vi "HC-SR04 Trigg Pulse.vi"(8 "Error In":errorcluster) -> (0 "Error Out":errorcluster)   [LabVIEW 2015]
uses:
  <vilib>/rvi/eio/common/nirviEmuTemplateMethod_errors.vi
  <vilib>/eio/EIONode/EIONode.xnode
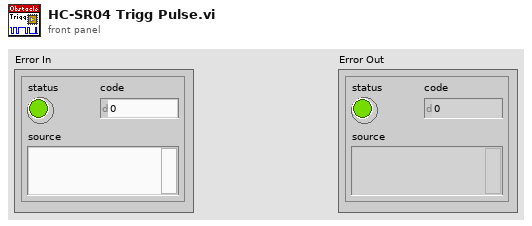
[diagram p1: front panel]
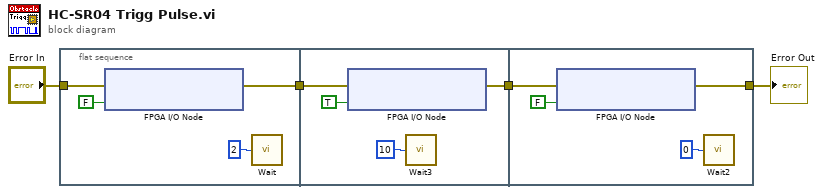
[diagram p0: block diagram]
diagram:
  n1 = flat-sequence {
    tunnel: [w6] -> w2
    tunnel: "Error In" -> [w5]
    tunnel: [w10] -> w3
    tunnel: w2 -> [w9]
    tunnel: [w14] -> w4
    tunnel: w3 -> [w13]
    frame #0 {
      n2 = xnode "FPGA I/O Node"("error in"=w5, "ConnectorA/DIO8"=FALSE) -> ("error out"=w6:errorcluster)  [unwired: 1 in, 1 out]
      n3 = call "Wait"("Count(uSec)"=i16 2) -> ()  [unwired: 1 out]
    }
    frame #1 {
      n4 = xnode "FPGA I/O Node"("error in"=w9, "ConnectorA/DIO8"=TRUE) -> ("error out"=w10:errorcluster)  [unwired: 1 in, 1 out]
      n5 = call "Wait3"("Count(uSec)"=i16 10) -> ()  [unwired: 1 out]
    }
    frame #2 {
      n6 = xnode "FPGA I/O Node"("error in"=w13, "ConnectorA/DIO8"=FALSE) -> ("error out"=w14:errorcluster)  [unwired: 1 in, 1 out]
      n7 = call "Wait2"("Count(uSec)"=i16 0) -> ()  [unwired: 1 out]
    }
  }
  "Error Out" <- w4
